vi "Write test data to file.vi"(0 "imei":string="ImeiImeiImeiIme", 1 "Meid":string="MediMeidMeidMe", 4 "SIM ID":string="SimSimSimSimSimSimID", 5 "Mac":string="MacMacMacMac", 7 "phone":string="ImeiImeiImeiIme", 9 "Serial Number":string="SerialNum", 11 "error in (no error)":errorcluster, 14 "Style":string="100060") -> (10 "PassFail":string="Fail", 15 "error out":errorcluster)   [LabVIEW 2013]
uses:
  Test Globals/Global 1.vi
  Main Support/Global 2.vi
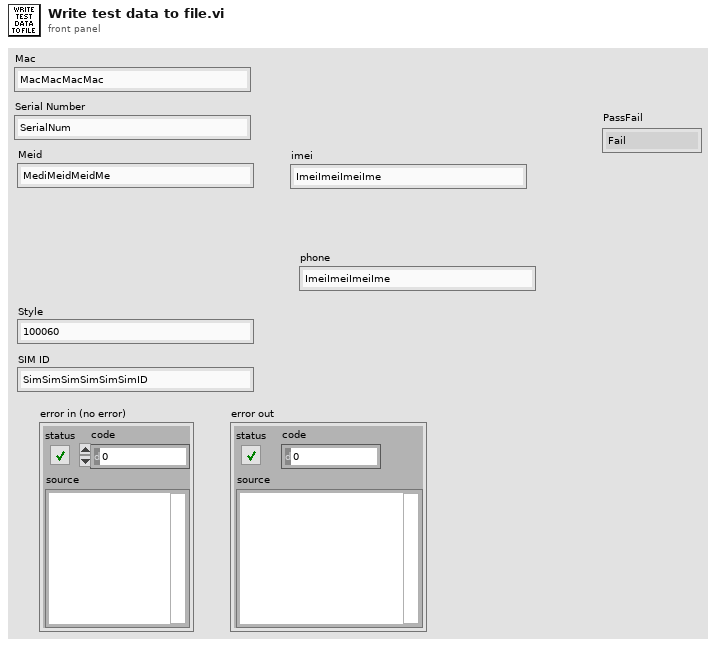
[diagram p1: front panel]
types:
  T1 = enum16{"get next serial available and assign", "change status to available"}
  T2 = cluster{"Test folder":string, "Top level":string, "Main":string, "Test report":string, "Work order qty":string, "Work order meid":string, "Work order imei":string, "Master meid imei list":string, "Master test data":string, "ZPL label info":string, "Pictures":string, "Setup info":string, "Work order":string, "Tests folder":string, "Tests steps folder":string, "Config folder":string, "Verizon Upload file":string, "Job data file":string, "Station globals":string, "Post test info":string}
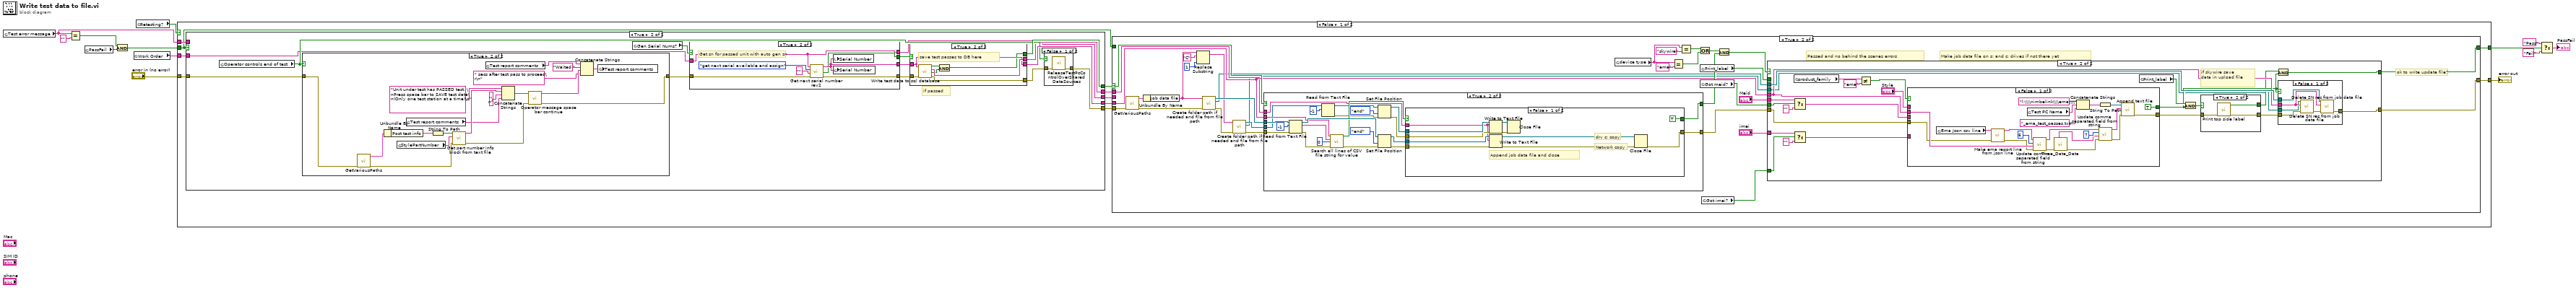
[diagram p0: block diagram]
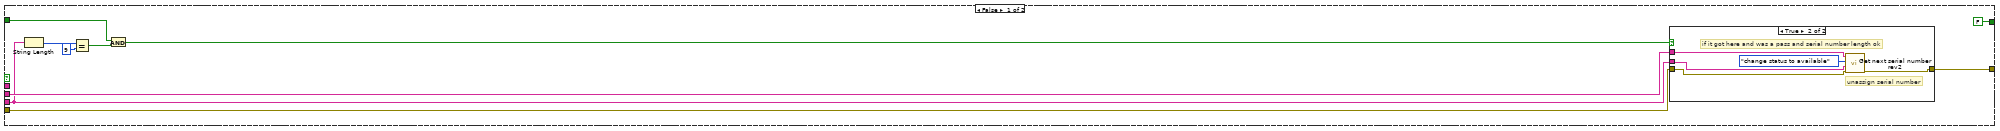
[diagram p2: hidden frame]
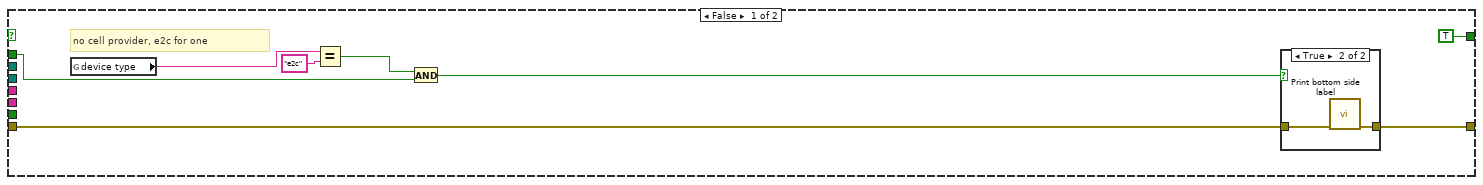
[diagram p4: hidden frame]
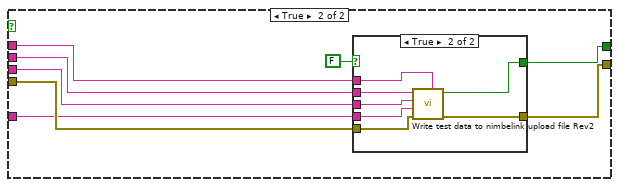
[diagram p6: hidden frame]
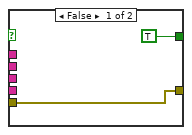
[diagram p7: hidden frame]
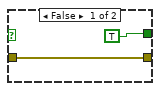
[diagram p8: hidden frame]
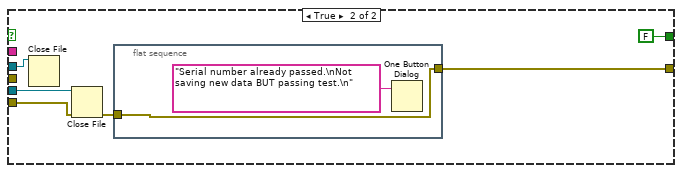
[diagram p11: hidden frame]
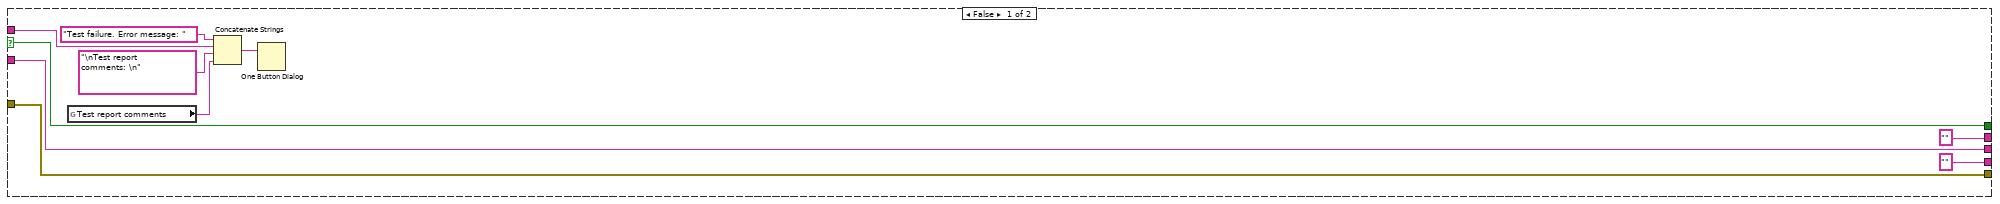
[diagram p12: hidden frame]
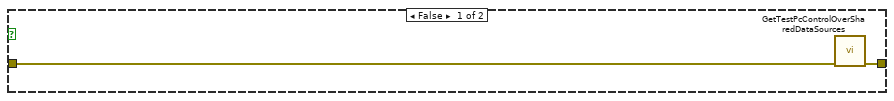
[diagram p14: hidden frame]
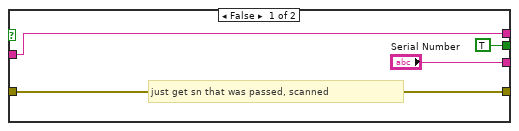
[diagram p15: hidden frame]
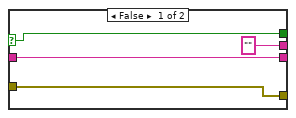
[diagram p16: hidden frame]
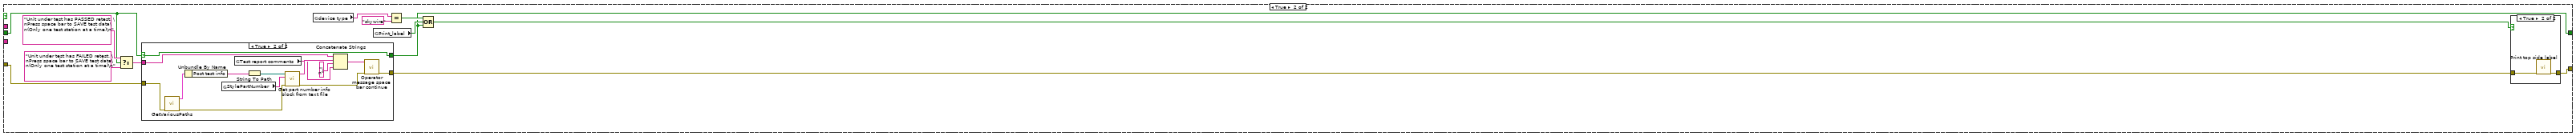
[diagram p17: hidden frame]
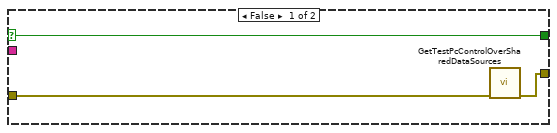
[diagram p18: hidden frame]
diagram:
  n1 = global read "Global 1.vi" "Test error message"() -> (w2:string)
  n2 = Equal?(x=w2, y="") -> (x = y?=w6:bool)
  n3 = global read "Global 2.vi" "PassFail"() -> (w5:bool)
  n4 = And(x=w6, y=w5) -> (x .and. y?=w3:bool)
  n5 = global read "Global 2.vi" "Work Order"() -> (w1:string)
  n6 = global read "Global 1.vi" "Retesting?"() -> (w8:bool)
  n7 = case shown="False" w8 {
    tunnel: [w24 w271] -> w10
    tunnel: [w23 w275] -> w9
    tunnel: "error in (no error)" -> [w18 w280]
    tunnel: w2 -> [w17 _]
    tunnel: w3 -> [w14 w274]
    tunnel: w1 -> [w16 _]
    frame False {
      n8 = case shown="True" w14 {
        selector: w14 -> [w208 _]
        tunnel: [w206 w216] -> w21
        tunnel: w18 -> [w206 w219]
        tunnel: [w208 w224] -> w22
        tunnel: w17 -> [w203 _]
        tunnel: ["" ("Serial number out") w220] -> w20
        tunnel: ["" ("Test rec csv line") w214] -> w19
        tunnel: w16 -> [w207 w212]
        tunnel: [w207 w211] -> w15
        frame False {
          n9 = global read "Global 1.vi" "Test report comments"() -> (w201:string)
          n10 = Concatenate Strings("Test failure. Error message: " ("string"), w203, "\nTest report comments: \n" ("string"), w201) -> (w205:string)
          n11 = One Button Dialog(message=w205) -> ()  [unwired: 1 in, 1 out]
        }
        frame True {
          # "if passed"
          n12 = global read "Global 2.vi" "Operator controls end of test"() -> (w215:bool)
          n13 = case shown="True" w215 {
            tunnel: w219 -> [w229 w239]
            tunnel: [w228 w235] -> w218
            frame False {
              n14 = call "GetTestPcControlOverSharedDataSources.vi"("error in (no error)"=w229) -> ("error out"=w228:errorcluster)  [unwired: 10 in]
            }
            frame True {
              n15 = call "GetVariousPaths.vi"("error in (no error)"=w239) -> ("error out"=w241:errorcluster, "Built Paths"=w247:T2)  [unwired: 9 in]
              n16 = Unbundle By Name(w247) -> ("Post test info"=w244:string)
              n17 = global read "Global 2.vi" "StylePartNumber"() -> (w242:string)
              n18 = global read "Global 1.vi" "Test report comments"() -> (w237:string)
              n19 = String To Path(string=w244) -> (path=w243:path)
              n20 = call "Get part number info block from text file.vi"("error in (no error)"=w241, "StylePartNum"=w242, "file (use dialog)"=w243) -> ("error out"=w236:errorcluster, "Info block"=w240:string)  [unwired: 6 in, 1 out]
              n21 = global read "Global 1.vi" "Test report comments"() -> (w234:string)
              n22 = Concatenate Strings("Unit under test has PASSED test. \nPress space bar to SAVE test data\n(Only one test station at a time)\n" ("Message"), w240, "\n" ("string"), w237) -> (w245:string)
              n23 = call "Operator message space bar continue.vi"("error in (no error)"=w236, "Message"=w245) -> ("error out"=w235:errorcluster, "Time waiting in secs"=w232:string)  [unwired: 8 in]
              n24 = Concatenate Strings(w234, "Waited " ("string"), w232, " secs after test pass to proceed\r\n" ("string")) -> (w230:string)
              n25 = global write "Global 1.vi" "Test report comments"(w230) -> ()
            }
          }
          n26 = global read "Global 1.vi" "Gen Serial Nums?"() -> (w222:bool)
          n27 = case shown="True" w222 {
            tunnel: w218 -> [w250 w255]
            tunnel: [w250 w258] -> w223
            tunnel: ["Serial Number" w256] -> w221
            tunnel: [TRUE ("Got serial number?") w254] -> w213
            tunnel: w212 -> [w248 w252]
            tunnel: [w248 w252] -> w211
            frame False {
              # "just get sn that was passed, scanned"
            }
            frame True {
              # "Get sn for passed unit with auto gen sn"
              n28 = call "Get next serial number rev2.vi"("Error in (no error)"=w255, "Serial number in"="", "Operation"=T1."get next serial available and assign", "Work order (WOXXXXX)"=w252) -> ("Error out"=w258:errorcluster, "OK?"=w254:bool, "Serial Number number out"=w256:string)  [unwired: 5 in]
              n29 = local write "Serial Number"(w256) -> ()
              n30 = global write "Global 2.vi" "Serial Number"(w256) -> ()
            }
          }
          n31 = case shown="True" w213 {
            selector: w213 -> [w262 _]
            tunnel: [w261 w267] -> w217
            tunnel: [w262 w263] -> w224
            tunnel: w223 -> [w261 w269]
            tunnel: w221 -> [w260 w266]
            tunnel: [w260 w266] -> w220
            tunnel: ["" ("Test rec csv line") w268] -> w214
            frame False {
            }
            frame True {
              # "save test passes to DB here"
              n32 = call "Write test data to sql database.vi"("error in (no error)"=w269, "Serial"=w266) -> ("error out"=w267:errorcluster, "No dup serial?"=w265:bool, "Test rec csv line"=w268:string, "Passed?"=w264:bool)  [unwired: 4 in]
              n33 = And(x=w264, y=w265) -> (x .and. y?=w263:bool)
            }
          }
          n34 = case shown="False" w215 {
            tunnel: w217 -> [w226 w227]
            tunnel: [w225 w227] -> w216
            frame False {
              n35 = call "ReleaseTestPcControlOverSharedDataSources.vi"("error in (no error)"=w226) -> ("error out"=w225:errorcluster)  [unwired: 10 in]
            }
            frame True {
            }
          }
        }
      }
      n36 = case shown="True" w22 {
        selector: w22 -> [_ w65]
        tunnel: [FALSE ("Write OK?") w70] -> w24
        tunnel: w21 -> [w32 w69]
        tunnel: [w31 w68] -> w23
        tunnel: w20 -> [w25 w64]
        tunnel: w19 -> [_ w55]
        tunnel: w15 -> [w33 _]
        tunnel: w14 -> [w30 _]
        frame False {
          n37 = String Length(string=w25) -> (length=w29:i32)
          n38 = Equal?(x=w29, y=9) -> (x = y?=w27:bool)
          n39 = And(x=w30, y=w27) -> (x .and. y?=w26:bool)
          n40 = case shown="True" w26 {
            tunnel: w33 -> [_ w39]
            tunnel: w25 -> [_ w38]
            tunnel: w32 -> [w35 w37]
            tunnel: [w35 w36] -> w31
            frame False {
            }
            frame True {
              # "if it got here and was a pass and serial number length ok"
              # "unassign serial number"
              n41 = call "Get next serial number rev2.vi"("Error in (no error)"=w37, "Serial number in"=w38, "Operation"=T1."change status to available", "Work order (WOXXXXX)"=w39) -> ("Error out"=w36:errorcluster)  [unwired: 5 in, 2 out]
            }
          }
        }
        frame True {
          # "Make job data file on s: and c: drives if not there yet"
          # "ok to write update file?"
          # "Passed and no behind the scenes errors"
          n42 = call "GetVariousPaths.vi"("error in (no error)"=w69) -> ("error out"=w54:errorcluster, "Built Paths"=w72:T2)  [unwired: 9 in]
          n43 = Unbundle By Name(w72) -> ("Job data file"=w53:string)
          n44 = Replace Substring(2:1 ("length (len. of substring)"), 4:"C" ("substring (\"\")"), 5:w53) -> (1:w50:string)  [unwired: 1 in, 1 out]
          n45 = call "Create folder path if needed and file from file path.vi"("error in"=w54, "String file path"=w53) -> ("error out"=w51:errorcluster, "file path"=w47:path, "New file refnum"=w52:refnum<file>)  [unwired: 7 in]
          n46 = call "Create folder path if needed and file from file path.vi"("error in"=w51, "String file path"=w50) -> ("error out"=w49:errorcluster, "file path"=w46:path, "New file refnum"=w48:refnum<file>)  [unwired: 7 in]
          n47 = case shown="True" w65 {
            selector: w65 -> [w157 _]
            tunnel: w52 -> [_ w175]
            tunnel: w64 -> [_ w171]
            tunnel: w49 -> [w158 w176]
            tunnel: [w158 w168] -> w71
            tunnel: [w157 w167] -> w66
            tunnel: w48 -> [_ w163]
            tunnel: w55 -> [_ w159]
            frame False {
            }
            frame True {
              n48 = Read from Text File(file (use dialog)=w175, count=-1, error in=w176) -> (refnum out=w179:refnum<file>, text=w172:string, error out=w174:errorcluster)  [unwired: 1 in, 1 out]
              n49 = Read from Text File(file (use dialog)=w163, count=-1) -> (refnum out=w166:refnum<file>, error out=w161:errorcluster)  [unwired: 2 in, 2 out]
              n50 = call "Search all lines of CSV file string for value.vi"("Compare value"=w171, "CSV file string"=w172, "CSV field (0-n)"=0, "error in"=w174) -> ("Found value"=w169:bool, "error out"=w173:errorcluster)  [unwired: 10 in]
              n51 = Set File Position(refnum=w166, from (0:start)=enum16{"start", "end", "current"}."end", error in=w161) -> (refnum out=w162:refnum<file>, error out=w160:errorcluster)  [unwired: 1 in]
              n52 = Set File Position(refnum=w179, from (0:start)=enum16{"start", "end", "current"}."end", error in=w173) -> (refnum out=w178:refnum<file>, error out=w177:errorcluster)  [unwired: 1 in]
              n53 = case shown="False" w169 {
                tunnel: w178 -> [w191 w197]
                tunnel: w177 -> [w192 w198]
                tunnel: [w190 w195] -> w168
                tunnel: [TRUE FALSE] -> w167
                tunnel: w162 -> [w184 w193]
                tunnel: w160 -> [w183 _]
                tunnel: w159 -> [w182 _]
                frame False {
                  # "Network copy"
                  # "drv c: copy"
                  # "Append job data file and close"
                  n54 = Write to Text File(file (use dialog)=w184, text=w182, error in=w183) -> (refnum out=w186:refnum<file>, error out=w185:errorcluster)  [unwired: 1 in, 1 out]
                  n55 = Write to Text File(file (use dialog)=w191, text=w182, error in=w192) -> (refnum out=w188:refnum<file>, error out=w189:errorcluster)  [unwired: 1 in, 1 out]
                  n56 = Close File(refnum=w186, error in=w185) -> ()  [unwired: 2 out]
                  n57 = Close File(refnum=w188, error in=w189) -> (error out=w190:errorcluster)  [unwired: 1 out]
                }
                frame True {
                  n58 = Close File(refnum=w193) -> ()  [unwired: 1 in, 2 out]
                  n59 = Close File(refnum=w197, error in=w198) -> (error out=w196:errorcluster)  [unwired: 1 out]
                  n60 = flat-sequence {
                    tunnel: w196 -> [w200]
                    tunnel: [w200] -> w195
                    frame #0 {
                      n61 = One Button Dialog(message="Serial number already passed.\nNot saving new data BUT passing test.\n") -> ()  [unwired: 1 in, 1 out]
                    }
                  }
                }
              }
            }
          }
          n62 = global read "Global 1.vi" "device type"() -> (w45:string)
          n63 = Equal?(x=w45, y="ema") -> (x = y?=w42:bool)
          n64 = Equal?(x=w45, y="skywire") -> (x = y?=w43:bool)
          n65 = Or(x=w43, y=w42) -> (x .or. y?=w41:bool)
          n66 = global read "Global 1.vi" "Print_label"() -> (w60:bool)
          n67 = global read "Global 1.vi" "Got meid?"() -> (w58:bool)
          n68 = global read "Global 1.vi" "Got imei?"() -> (w61:bool)
          n69 = And(x=w41, y=w66) -> (x .and. y?=w67:bool)
          n70 = case shown="True" w67 {
            tunnel: w71 -> [w75 w107]
            tunnel: [w74 w106] -> w68
            tunnel: w64 -> [_ w104]
            tunnel: [TRUE ("Write OK?") w89] -> w70
            tunnel: w47 -> [_ w105]
            tunnel: "Meid" -> [_ w97]
            tunnel: "imei" -> [_ w94]
            tunnel: w61 -> [_ w93]
            tunnel: w60 -> [w73 _]
            tunnel: w58 -> [_ w88]
            tunnel: w46 -> [_ w87]
            frame False {
              # "no cell provider, e2c for one"
              n71 = global read "Global 1.vi" "device type"() -> (w79:string)
              n72 = Equal?(x=w79, y="e2c") -> (x = y?=w77:bool)
              n73 = And(x=w77, y=w73) -> (x .and. y?=w76:bool)
              n74 = case shown="True" w76 {
                tunnel: w75 -> [w81 w83]
                tunnel: [w81 w82] -> w74
                frame False {
                }
                frame True {
                  n75 = call "Print bottom side label.vi"("error in (no error)"=w83) -> ("error out"=w82:errorcluster)  [unwired: 7 in, 1 out]
                }
              }
            }
            frame True {
              # "if skywire save\ndata in upload file"
              n76 = Select(t=w97, s=w88, f="") -> (s? t:f=w96:string)
              n77 = Select(t=w94, s=w93, f="") -> (s? t:f=w92:string)
              n78 = global read "Global 1.vi" "product_family"() -> (w86:string)
              n79 = Not Equal?(x=w86, y="ema") -> (x != y?=w84:bool)
              n80 = case shown="False" w84 {
                tunnel: w107 -> [w114 w135]
                tunnel: w104 -> [w124 w134]
                tunnel: [w127 w133] -> w101
                tunnel: "Style" -> [_ w132]
                tunnel: w96 -> [_ w131]
                tunnel: w92 -> [_ w130]
                tunnel: [TRUE ("Write OK?") w129] -> w91
                frame False {
                  n81 = global read "Global 1.vi" "Ema Json csv line"() -> (w116:string)
                  n82 = call "Make ema report line from json line.vi"("error in (no error)"=w114, "Ema Json csv line"=w116) -> ("error out"=w113:errorcluster, "EMA report file line"=w115:string)  [unwired: 8 in]
                  n83 = global read "Global 1.vi" "Test PC Name"() -> (w112:string)
                  n84 = call "Update comma separated field from string.vi"("error in (no error)"=w113, "New field data"=w124, "Field number (1-n)"=u32 6, "CSV string with field to update"=w115) -> ("error out"=w120:errorcluster, "Updated csv string"=w123:string)  [unwired: 6 in]
                  n85 = call "Time_Date_Data.vi"("error in (no error)"=w120) -> ("error out"=w119:errorcluster, "EMA time"=w117:string)  [unwired: 3 in, 6 out]
                  n86 = Concatenate Strings("l:\\\\nimbelink\\\\ema\\\\" ("string"), w112, "_ema_test_passes.txt" ("string")) -> (w109:string)
                  n87 = String To Path(string=w109) -> (path=w108:path)
                  n88 = call "Update comma separated field from string.vi"("error in (no error)"=w119, "New field data"=w117, "Field number (1-n)"=u32 7, "CSV string with field to update"=w123) -> ("error out"=w118:errorcluster, "Updated csv string"=w121:string)  [unwired: 6 in]
                  n89 = call "Append text file.vi"("error in"=w118, "text to write"=w121, "file path (use dialog)"=w108) -> ("error out"=w127:errorcluster)  [unwired: 8 in]
                }
                frame True {
                  n90 = case shown="True" FALSE {
                    tunnel: w135 -> [w137 w144]
                    tunnel: w134 -> [_ w143]
                    tunnel: [w137 w142] -> w133
                    tunnel: w132 -> [_ w141]
                    tunnel: w131 -> [_ w140]
                    tunnel: w130 -> [_ w139]
                    tunnel: [TRUE ("Write OK?") w138] -> w129
                    frame False {
                    }
                    frame True {
                      n91 = call "Write test data to nimbelink upload file Rev2.vi"("Style"=w141, "error in (no error)"=w144, "imei"=w139, "Meid"=w140, "Serial Number"=w143) -> ("error out"=w142:errorcluster, "Write OK?"=w138:bool)  [unwired: 2 in, 1 out]
                    }
                  }
                }
              }
              n92 = global read "Global 1.vi" "Print_label"() -> (w103:bool)
              n93 = And(x=w103, y=w91) -> (x .and. y?=w102:bool)
              n94 = case shown="True" w102 {
                tunnel: w101 -> [w146 w149]
                tunnel: [w146 w148] -> w100
                tunnel: [TRUE ("Print Label OK?") w147] -> w90
                frame False {
                }
                frame True {
                  n95 = call "Print top side label.vi"("error in (no error)"=w149) -> ("error out"=w148:errorcluster, "Print Label OK?"=w147:bool)  [unwired: 7 in]
                }
              }
              n96 = And(x=w90, y=w91) -> (x .and. y?=w89:bool)
              n97 = case shown="False" w91 {
                tunnel: w100 -> [w155 w156]
                tunnel: [w152 w156] -> w106
                tunnel: w105 -> [w151 _]
                tunnel: w104 -> [w154 _]
                tunnel: w87 -> [w150 _]
                frame False {
                  n98 = call "Delete SN rec from job data file.vi"("error in"=w155, "Serial number"=w154, "file (use dialog)"=w150) -> ("error out"=w153:errorcluster)  [unwired: 8 in]
                  n99 = call "Delete SN rec from job data file.vi"("error in"=w153, "Serial number"=w154, "file (use dialog)"=w151) -> ("error out"=w152:errorcluster)  [unwired: 8 in]
                }
                frame True {
                }
              }
            }
          }
        }
      }
    }
    frame True {
      n100 = Select(t="Unit under test has PASSED retest. \nPress space bar to SAVE test data\n(Only one test station at a time)\n" ("Message"), s=w274, f="Unit under test has FAILED retest. \nPress space bar to SAVE test data\n(Only one test station at a time)\n" ("Message")) -> (s? t:f=w276:string)
      n101 = case shown="True" w274 {
        selector: w274 -> [w283 w286]
        tunnel: w280 -> [w285 w291]
        tunnel: [w284 w290] -> w279
        tunnel: w276 -> [_ w287]
        tunnel: [w283 w286] -> w271
        frame False {
          n102 = call "GetTestPcControlOverSharedDataSources.vi"("error in (no error)"=w285) -> ("error out"=w284:errorcluster)  [unwired: 10 in]
        }
        frame True {
          n103 = call "GetVariousPaths.vi"("error in (no error)"=w291) -> ("error out"=w294:errorcluster, "Built Paths"=w299:T2)  [unwired: 9 in]
          n104 = Unbundle By Name(w299) -> ("Post test info"=w297:string)
          n105 = global read "Global 2.vi" "StylePartNumber"() -> (w295:string)
          n106 = global read "Global 1.vi" "Test report comments"() -> (w288:string)
          n107 = String To Path(string=w297) -> (path=w296:path)
          n108 = call "Get part number info block from text file.vi"("error in (no error)"=w294, "StylePartNum"=w295, "file (use dialog)"=w296) -> ("error out"=w293:errorcluster, "Info block"=w292:string)  [unwired: 6 in, 1 out]
          n109 = Concatenate Strings(w287, w292, "\n" ("string"), w288) -> (w298:string)
          n110 = call "Operator message space bar continue.vi"("error in (no error)"=w293, "Message"=w298) -> ("error out"=w290:errorcluster)  [unwired: 8 in, 1 out]
        }
      }
      n111 = global read "Global 1.vi" "device type"() -> (w281:string)
      n112 = global read "Global 1.vi" "Print_label"() -> (w272:bool)
      n113 = Equal?(x=w281, y="skywire") -> (x = y?=w273:bool)
      n114 = Compound Arithmetic op=OR(w273, w272, w271) -> (w270:bool)
      n115 = case shown="True" w270 {
        tunnel: w279 -> [w300 w302]
        tunnel: [w300 w301] -> w275
        frame False {
        }
        frame True {
          n116 = call "Print top side label.vi"("error in (no error)"=w302) -> ("error out"=w301:errorcluster)  [unwired: 7 in, 1 out]
        }
      }
    }
  }
  "error out" <- w9
  n117 = Select(t="Pass", s=w10, f="Fail") -> (s? t:f=→"PassFail":string)
